vi "Is Circle-Rect Collision.vi"(1 "Other Collider in":refnum<class "Rect Collider.lvclass">, 2 "Other Object in":refnum<class "SimulationObject.lvclass">, 3 "Self Collider in":refnum<class "Circle Collider.lvclass">, 4 "Self Object in":refnum<class "SimulationObject.lvclass">) -> (0 "Are Colliding":bool)   [LabVIEW 2022 SP3, in "Circle Collider.lvclass"]
uses:
  Circle Collider.lvclass
  SimulationObject/SimulationObject.lvclass
  Rect Collider/Rect Collider.lvclass
  SimulationObject/SimulationObject.lvclass/SimulationObject.ctl
  Components/Transform/Transform.lvclass/Transform.ctl
  Math/Vector2/Vector2.lvclass/Vector2.ctl
  Circle Collider.lvclass/Circle Collider.ctl
  Rect Collider/Rect Collider.lvclass/Rect Collider.ctl
  Rect Collider/Read Width.vi
  Rect Collider/Read Height.vi
  Read Radius.vi
  Math/Vector2/Read x.vi
  Math/Vector2/Read y.vi
  Components/Transform/Transform.lvclass
  Math/Vector2/Vector2.lvclass
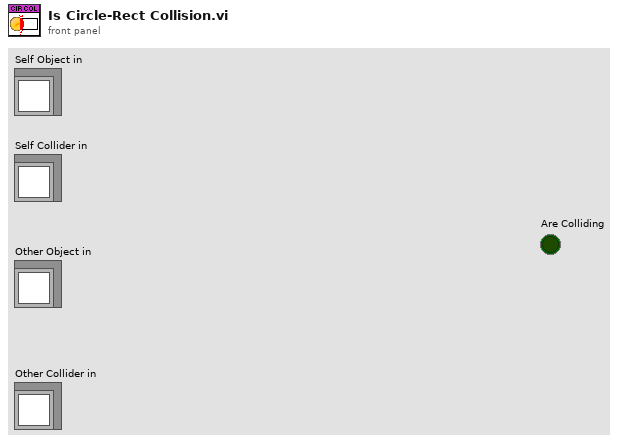
[diagram p1: front panel]
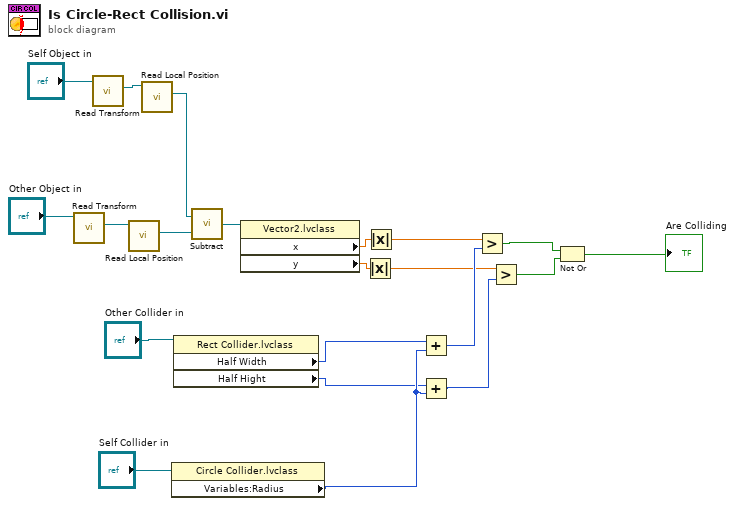
[diagram p0: block diagram]
diagram:
  n1 = call "Read Transform.vi"("SimulationObject in"="Other Object in") -> ("Transform out"=w19:refnum<class "Transform.lvclass">)  [unwired: 8 in, 2 out]
  n2 = call "Read Transform.vi"("SimulationObject in"="Self Object in") -> ("Transform out"=w17:refnum<class "Transform.lvclass">)  [unwired: 8 in, 2 out]
  n3 = call "Read Local Position.vi"("Transform in"=w19) -> ("Local Position out"=w15:refnum<class "Vector2.lvclass">)  [unwired: 8 in, 2 out]
  n4 = call "Read Local Position.vi"("Transform in"=w17) -> ("Local Position out"=w14:refnum<class "Vector2.lvclass">)  [unwired: 8 in, 2 out]
  n5 = property class="Circle Collider.lvclass"(reference="Self Collider in") -> ("Variables:Radius"=w9:i16)  [unwired: 1 in, 2 out]
  n6 = property class="Rect Collider.lvclass"(reference="Other Collider in") -> ("Half Width"=w1:i16, "Half Hight"=w2:i16)  [unwired: 1 in, 2 out]
  n7 = call "Subtract.vi"("Vec2 b in"=w15, "Vec2 a in"=w14) -> ("Vec2 out"=w13:refnum<class "Vector2.lvclass">)
  n8 = property class="Vector2.lvclass"(reference=w13) -> ("x"=w12:sgl, "y"=w11:sgl)  [unwired: 1 in, 2 out]
  n9 = Absolute Value(x=w11) -> (abs(x)=w7:sgl)
  n10 = Absolute Value(x=w12) -> (abs(x)=w10:sgl)
  n11 = Add(x=w1, y=w9) -> (x+y=w8:i16)
  n12 = Add(x=w2, y=w9) -> (x+y=w6:i16)
  n13 = Greater?(x=w10, y=w8) -> (0:w5:bool)
  n14 = Greater?(x=w7, y=w6) -> (0:w4:bool)
  n15 = Not Or(1:w4, 2:w5) -> (0:→"Are Colliding":bool)
